vi "StandardInit.vi"(1 "Incoming Handle":i32) -> (0 "Outgoing Handle":i32)   [LabVIEW 2019]
uses:
  Madlib.dll
panel:
  # "This VI implements an initialization sequence for use with \na single Nano-Drive."
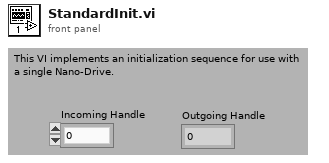
[diagram p1: front panel]
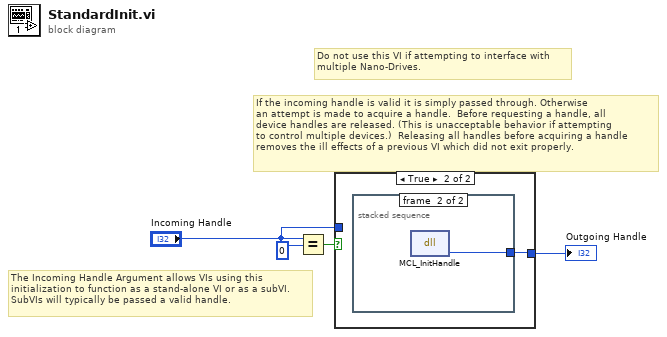
[diagram p0: block diagram]
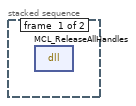
[diagram p3: hidden frame]
diagram:
  # "The Incoming Handle Argument allows VIs using this\ninitialization to function as a stand-alone VI or as a subVI.\nSubVIs will typically be passed a valid handle."
  # "Do not use this VI if attempting to interface with\nmultiple Nano-Drives."
  # "If the incoming handle is valid it is simply passed through. Otherwise\nan attempt is made to acquire a handle.  Before requesting a handle, all\ndevice handles are released. (This is unacceptable behavior if attempting\nto control multiple devices.)  Releasing all handles before acquiring a handle\nremoves the ill effects of a previous VI which did not exit properly."
  n1 = Equal?(x="Incoming Handle", y=0) -> (x = y?=w3:bool)
  n2 = case shown="True" w3 {
    tunnel: [w5 w6] -> w1
    tunnel: "Incoming Handle" -> [w5 _]
    frame False {
    }
    frame True {
      n3 = stacked-sequence {
        tunnel: [_ w7] -> w6
        frame #0 {
          n4 = dll-call lib="C:/Users/admin/Desktop/controller/SubVIs_nanostage/MADLib.dll" fn="MCL_ReleaseAllHandles"() -> ()  [unwired: 4 in, 2 out]
        }
        frame #1 {
          n5 = dll-call lib="C:/Users/admin/Desktop/controller/SubVIs_nanostage/MADLib.dll" fn="MCL_InitHandle"() -> (w7:i32)  [unwired: 3 in, 2 out]
        }
      }
    }
  }
  "Outgoing Handle" <- w1
